vi "Handle Value Change.vi"(5 "VolatusAPI":refnum<class "VolatusAPI.lvclass">, 7 "CtlRef":refnum<vi>, 8 "error in (no error)":errorcluster, 9 "NewVal":variant, 10 "OldVal":variant, 11 "OnValueChangeHandler in":refnum<class "OnValueChangeHandler.lvclass">) -> (0 "error out":errorcluster, 3 "OnValueChangeHandler out":refnum<class "OnValueChangeHandler.lvclass">)   [LabVIEW 2020, in "VolatusGUI.lvlib" / "OnValueChangeHandler.lvclass"]
uses:
  OnValueChangeHandler.lvclass
  Volatus/VolatusAPI/VolatusAPI.lvclass
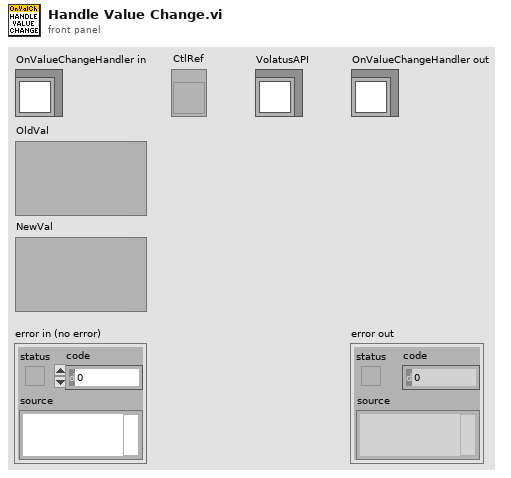
[diagram p1: front panel]
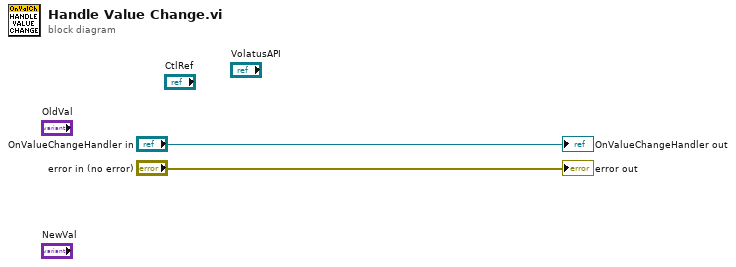
[diagram p0: block diagram]
diagram:
  "error out" <- "error in (no error)"
  "OnValueChangeHandler out" <- "OnValueChangeHandler in"
